vi "CALC_FUNC_DOM_USER_RANG.vi"(0 "VISA IN":refnum<visa-resource-name>, 1 "Range number":i32, 5 "error in":errorcluster, 7 "Channel":i32) -> (14 "VISA Out":refnum<visa-resource-name>, 19 "error out":errorcluster)   [LabVIEW 2018, in "PNA-X.lvlib"]
doc: "CALCulate<cnum>:FUNCtion:DOMain:USER[:RANGe] <range> \n1516\n\n(Read-Write) Sets the range used to calculate trace statistics. Each channel has 16 user ranges. The xaxis \nrange is specified with the CALC:FUNC:DOM:USER:START and STOP commands. \nSee Critical Note \nParameters \n<cnum> Channel number of the measurement. There must be a selected measurement \non that channel. If unspecified, <cnum> is set to 1. \n<range> Range number. Choose from: 0 to 16 \n0 is Full Span of the current x-axis range \n1 to 16 are user-specified ranges \nExamples CALC:FUNC:DOM:USER 4 \ncalculate2:function:domain:user:range 0 \nQuery Syntax CALCulate<cnum>:FUNCtion:DOMain:USER[:RANGe]? \nReturn Type Numeric \nDefault 0 - Full Span"
uses:
  PNA-X.lvlib
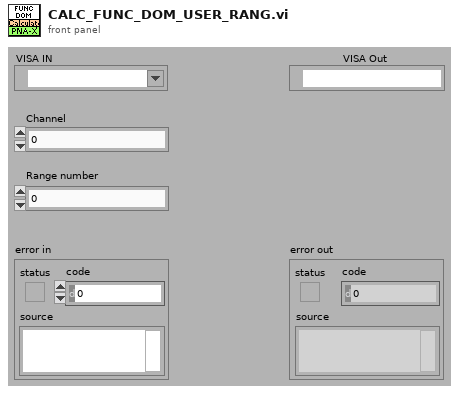
[diagram p1: front panel]
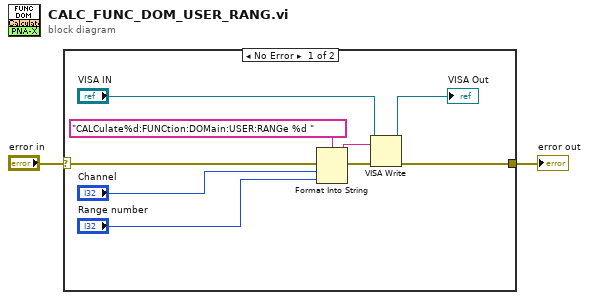
[diagram p0: block diagram]
diagram:
  n1 = case shown="No Error" "error in" {
    selector: "error in" -> [w11 w12]
    tunnel: [w6 w12] -> w1
    frame No Error {
      n2 = Format Into String(format string="CALCulate%d:FUNCtion:DOMain:USER:RANGe %d " ("Cmdline"), error in=w11, "Channel", "Range number") -> (resulting string=w9:string, error out=w10:errorcluster)  [unwired: 1 in]
      n3 = VISA Write(VISA resource name="VISA IN", write buffer=w9, error in (no error)=w10) -> (VISA resource name out=→"VISA Out":refnum<visa-resource-name>, error out=w6:errorcluster)  [unwired: 1 out]
    }
    frame Error {
    }
  }
  "error out" <- w1
